vi "obj_DataLog Tag Expression Evaluator.vi"(0 "method":T1, 5 "variable":string, 7 "value in":dbl, 9 "expression/scriptlet":string, 11 "error in (no error)":errorcluster) -> (8 "value out":dbl, 15 "error out":errorcluster)   [LabVIEW 2012]
doc: "Allows evaluation of expressions that can include tag names as variables. For set&hold and sample tags, these variables are set to their current value (the value of the last written point).\n\nThis \"object\" caches variables and parsed expressions for fast evaluation and assignment. It is possible to {set} or {get} a variable, {eval}uate an expression, or evaluate and {assign} an expression to a variable. The {isvalid} method tests whether a variable name is a valid identifier and does not collide with one of the predefined functions or numbers. To set initial values or define custom functions, {execute} a scriptlet. Finally, all custom variables and functions can be {clear}ed.\n\nExpressions and scriptlets can make use Lua's arithmetic operators, the predefined numerical values \"pi\", \"_NaN\", and \"_Inf\", the functions in the math library (sin(), sqrt(), etc.) and the lv library functions for bitwise and other integer operations (andU32(), addI8(), etc.). To promote compact expressions, both sets of functions are available only without their library (\"math.\", \"lv.\") table prefix."
uses:
  typedefs/t_DataLog Tag Expression Evaluator Methods.ctl
  luaview/typedefs/t_LuaVIEW Reference.ctl
  luaview/subvis/private/LuaVIEW Push (string).vi
  luaview/subvis/private/LuaVIEW Push (number).vi
  luaview/subvis/private/LuaVIEW Pull (number).vi
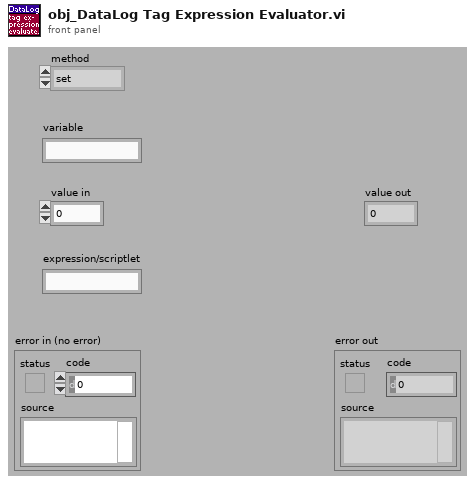
[diagram p1: front panel]
types:
  T1 = typedef "t_DataLog Tag Expression Evaluator Methods.ctl" = enum16{"set", "get", "eval", "assign", "execute", "isvalid", "clear"}
  T2 = typedef "t_LuaVIEW Reference.ctl" = refnum<k1>
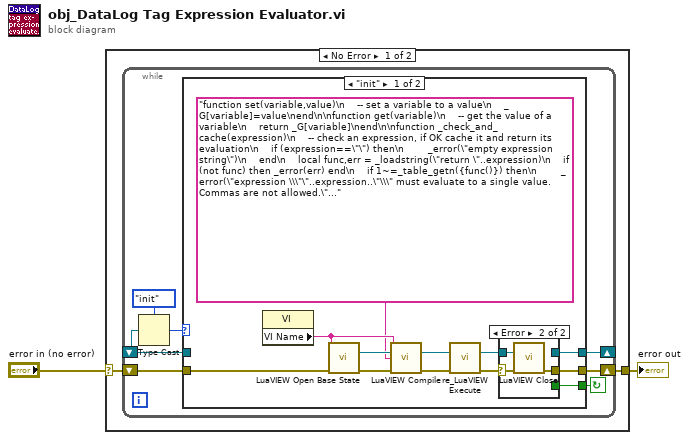
[diagram p0: block diagram]
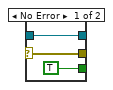
[diagram p2: hidden frame]
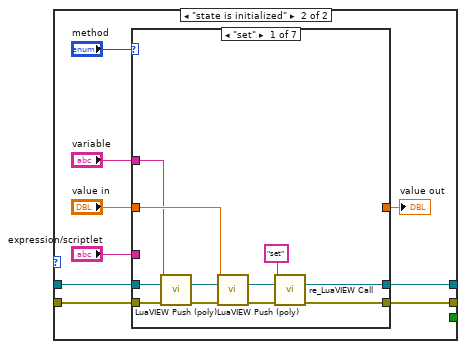
[diagram p3: hidden frame]
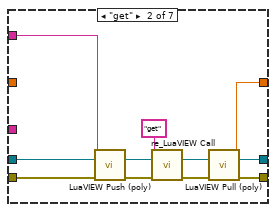
[diagram p4: hidden frame]
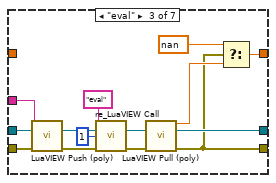
[diagram p5: hidden frame]
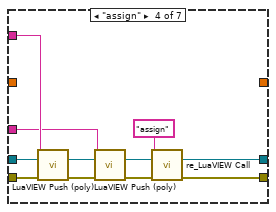
[diagram p6: hidden frame]
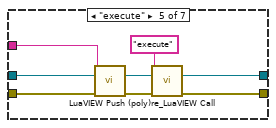
[diagram p7: hidden frame]
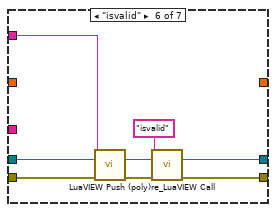
[diagram p8: hidden frame]
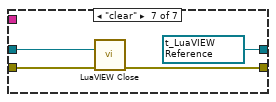
[diagram p9: hidden frame]
diagram:
  n1 = case shown="No Error" "error in (no error)" {
    selector: "error in (no error)" -> [w3 w106]
    tunnel: [w4 w106] -> w1
    frame No Error {
      n2 = while {
        shift-right: [w10] -> _
        shift-left: _ -> [w8]
        shift-right: [w9] -> w4
        shift-left: w3 -> [w11]
        stop <- w5 continue-if-true
        n3 = Type Cast(type=enum32{"init", "state is initialized"}."init", x=w8) -> (*(type *) &x=w6:enum32{"init", "state is initialized"})
        n4 = case shown="\"init\"" w6 {
          tunnel: w11 -> [w23 w38]
          tunnel: [w14 w35] -> w10
          tunnel: [w16 w36] -> w9
          tunnel: w8 -> [_ w37]
          tunnel: [w12 _] -> w5
          frame "init" {
            n5 = property class="VI"() -> ("VI Name"=w19:string)  [unwired: 2 in, 2 out]
            n6 = call "LuaVIEW Open Base State.vi"("close identifier (none)"=w19, "error in (no error)"=w23) -> ("LuaVIEW reference"=w21:T2, "error out"=w17:errorcluster)  [unwired: 12 in]
            n7 = call "LuaVIEW Compile.vi"("script name"=w19, "LuaVIEW reference in"=w21, "script"="function set(variable,value)\n    -- set a variable to a value\n    _G[variable]=value\nend\n\nfunction get(variable)\n    -- get the value of a variable\n    return _G[variable]\nend\n\nfunction _check_and_cache(expression)\n    -- check an expression, if OK cache it and return its evaluation\n    if (expression==\"\") then\n        _error(\"empty expression string\")\n    end\n    local func,err = _loadstring(\"return \"..expression)\n    if (not func) then _error(err) end\n    if 1~=_table_getn({func()}) then\n        _error(\"expression \\\"\"..expression..\"\\\" must evaluate to a single value. Commas are not allowed.\")\n    end\n    local result=func()\n    if _type(result)~=\"number\" then\n        _error(\"expression \\\"\"..expression..\"\\\" does not evaluate to a number\")\n    end\n    _expression_cache[expression]=func\n    return result\nend\n\nfunction eval(expression)\n    -- evaluate an expression and return its value\n    local func=_expression_cache[expression]\n    if (func) then\n        -- expression already parsed and cached\n        return func()\n    end\n    return _check_and_cache(expression)\nend\n\nfunction assign(variable,expression)\n    -- evaluate an expression and assign it to a variable\n    local func=_expression_cache[expression]\n    if (func) then\n        -- expression already parsed and cached\n        _G[variable]=func()\n        return\n    end\n    _G[variable]=_check_and_cache(expression)\nend\n\nfunction execute(statements)\n    -- execute statements, e.g. setting initial variable values\n    -- or defining custom functions\n    local func,err=_loadstring(statements)\n    if (not func) then\n        _error(err)\n    end\n    func()\nend\n\nfunction isvalid(variable)\n    -- check if a variable name is valid for assignment\n    if _name_reserved[variable] then\n        _error(\"\\\"\"..variable..\"\\\" is not a valid variable name: it is reserved for a predefined \".._type(_G[variable]))\n    end\n    if _string_find(variable,\"[^_%w]\") then\n        _error(\"\\\"\"..variable..\"\\\" is not a valid variable name: only underscores and alphanumerical characters are allowed.\")\n    end\n    if (not _loadstring(\"return {\"..variable..\"=42}\")) then\n        _error(\"\\\"\"..variable..\"\\\" is not a valid variable name: leading digits and Lua reserved names are prohibited.\")\n    end    \nend\n\n--start with an empty expression cache\n_expression_cache={}\n\n-- hide functions and tables that do not belong in expressions\n_error=error\n_type=type\n_table_getn=table.getn\n_string_find=string.find\n_loadstring=loadstring\nretain={\nretain=true,\nset=true,\nget=true,\neval=true,\nassign=true,\nexecute=true,\nisvalid=true,\nstring=true,\nmath=true,\n}\nfor k,v in pairs(lv) do\n    if (string.find(k,\"I8\") or string.find(k,\"U8\") or string.find(k,\"I16\") or string.find(k,\"U16\") or string.find(k,\"I32\") or string.find(k,\"U32\")) then\n        _G[k]=v\n        retain[k]=true\n    end\nend\n_name_reserved={}\nfor k,v in pairs(_G) do\n    if _type(k)==\"string\" and not (retain[k] or math[k] or string.sub(k,1,1)==\"_\") then\n        _G[k]=nil\n    else\n        _name_reserved[k]=true\n    end\nend\nmath=nil\n_name_reserved.math=nil\nretain=nil\n_name_reserved.retain=nil\nstring=nil\n_name_reserved.string=nil\n", "error in (no error)"=w17) -> ("LuaVIEW reference out"=w20:T2, "error out"=w22:errorcluster)  [unwired: 10 in]
            n8 = call "re_LuaVIEW Execute.vi"("LuaVIEW reference in"=w20, "error in (no error)"=w22) -> ("LuaVIEW reference out"=w15:T2, "error out"=w13:errorcluster)  [unwired: 12 in]
            n9 = case shown="Error" w13 {
              selector: w13 -> [w25 w29]
              tunnel: w15 -> [w26 w28]
              tunnel: [w25 w27] -> w16
              tunnel: [w26 _] -> w14
              tunnel: [TRUE _] -> w12
              frame No Error {
              }
              frame Error {
                n10 = call "LuaVIEW Close.vi"("LuaVIEW reference"=w28, "error in (no error)"=w29) -> ("dup error"=w27:errorcluster)  [unwired: 13 in]
              }
            }
          }
          frame "state is initialized" {
            n11 = case shown="\"set\"" "method" {
              tunnel: w38 -> [w46 w50 w66 w82 w89 w96 w104]
              tunnel: w37 -> [w47 w51 w67 w83 w90 w97 w105]
              tunnel: [w39 w60 w61 w75 w87 w94 w103] -> w36
              tunnel: [w40 w55 w70 w76 w88 w95 w102] -> w35
              tunnel: "expression/scriptlet" -> [_ _ w68 w77 w86 _ _]
              tunnel: "value in" -> [w42 _ _ _ _ _ _]
              tunnel: "variable" -> [w41 w52 _ w78 _ w98 _]
              tunnel: [_ w54 w64 _ _ _ _] -> w30
              frame "set" {
                n12 = call-poly "LuaVIEW Push (poly).vi"("string"=w41, "LuaVIEW reference in"=w47, "error in (no error)"=w46) -> ("LuaVIEW reference out"=w44:T2, "error out"=w45:errorcluster)  [unwired: 11 in]
                n13 = call-poly "LuaVIEW Push (poly).vi"("number"=w42, "LuaVIEW reference in"=w44, "error in (no error)"=w45) -> ("LuaVIEW reference out"=w48:T2, "error out"=w49:errorcluster)  [unwired: 11 in]
                n14 = call "re_LuaVIEW Call.vi"("function name"="set", "LuaVIEW reference in"=w48, "error in (no error)"=w49) -> ("LuaVIEW reference out"=w40:T2, "error out"=w39:errorcluster)  [unwired: 11 in]
              }
              frame "get" {
                n15 = call-poly "LuaVIEW Push (poly).vi"("string"=w52, "LuaVIEW reference in"=w51, "error in (no error)"=w50) -> ("LuaVIEW reference out"=w58:T2, "error out"=w59:errorcluster)  [unwired: 11 in]
                n16 = call "re_LuaVIEW Call.vi"("function name"="get", "LuaVIEW reference in"=w58, "error in (no error)"=w59) -> ("LuaVIEW reference out"=w56:T2, "error out"=w57:errorcluster)  [unwired: 11 in]
                n17 = call-poly "LuaVIEW Pull (poly).vi"("LuaVIEW reference in"=w56, "error in (no error)"=w57) -> ("number"=w54:dbl, "LuaVIEW reference out"=w55:T2, "error out"=w60:errorcluster)  [unwired: 11 in]
              }
              frame "eval" {
                n18 = call-poly "LuaVIEW Push (poly).vi"("string"=w68, "LuaVIEW reference in"=w67, "error in (no error)"=w66) -> ("LuaVIEW reference out"=w73:T2, "error out"=w74:errorcluster)  [unwired: 11 in]
                n19 = call "re_LuaVIEW Call.vi"("function name"="eval", "LuaVIEW reference in"=w73, "required results (no checking needed)"=1, "error in (no error)"=w74) -> ("LuaVIEW reference out"=w71:T2, "error out"=w72:errorcluster)  [unwired: 10 in]
                n20 = call-poly "LuaVIEW Pull (poly).vi"("LuaVIEW reference in"=w71, "error in (no error)"=w72) -> ("number"=w63:dbl, "LuaVIEW reference out"=w70:T2, "error out"=w61:errorcluster)  [unwired: 11 in]
                n21 = Select(t=nan, s=w61, f=w63) -> (s? t:f=w64:dbl)
              }
              frame "assign" {
                n22 = call-poly "LuaVIEW Push (poly).vi"("string"=w78, "LuaVIEW reference in"=w83, "error in (no error)"=w82) -> ("LuaVIEW reference out"=w80:T2, "error out"=w81:errorcluster)  [unwired: 11 in]
                n23 = call-poly "LuaVIEW Push (poly).vi"("string"=w77, "LuaVIEW reference in"=w80, "error in (no error)"=w81) -> ("LuaVIEW reference out"=w84:T2, "error out"=w85:errorcluster)  [unwired: 11 in]
                n24 = call "re_LuaVIEW Call.vi"("function name"="assign", "LuaVIEW reference in"=w84, "error in (no error)"=w85) -> ("LuaVIEW reference out"=w76:T2, "error out"=w75:errorcluster)  [unwired: 11 in]
              }
              frame "execute" {
                n25 = call-poly "LuaVIEW Push (poly).vi"("string"=w86, "LuaVIEW reference in"=w90, "error in (no error)"=w89) -> ("LuaVIEW reference out"=w92:T2, "error out"=w93:errorcluster)  [unwired: 11 in]
                n26 = call "re_LuaVIEW Call.vi"("function name"="execute", "LuaVIEW reference in"=w92, "error in (no error)"=w93) -> ("LuaVIEW reference out"=w88:T2, "error out"=w87:errorcluster)  [unwired: 11 in]
              }
              frame "isvalid" {
                n27 = call-poly "LuaVIEW Push (poly).vi"("string"=w98, "LuaVIEW reference in"=w97, "error in (no error)"=w96) -> ("LuaVIEW reference out"=w100:T2, "error out"=w101:errorcluster)  [unwired: 11 in]
                n28 = call "re_LuaVIEW Call.vi"("function name"="isvalid", "LuaVIEW reference in"=w100, "error in (no error)"=w101) -> ("LuaVIEW reference out"=w95:T2, "error out"=w94:errorcluster)  [unwired: 11 in]
              }
              frame "clear" {
                w102 = T2 refnum items=["LuaVIEW"] ("LuaVIEW reference out")
                n29 = call "LuaVIEW Close.vi"("LuaVIEW reference"=w105, "error in (no error)"=w104) -> ("dup error"=w103:errorcluster)  [unwired: 13 in]
              }
            }
            "value out" <- w30
          }
        }
      }
    }
    frame Error {
    }
  }
  "error out" <- w1
